vi "Disabled.vi"(11 "Call Context":T1) -> ()   [LabVIEW 2013]
doc: "This VI is called each time a disabled packet is received from the DS. It is often used to prepare for the next robot mode, to calibrate sensors, etc."
uses:
  <vilib>/Rock Robotics/WPI/DriverStation/WPI_DriverStationDerivedRobotMode.ctl
  Robot Global Data.vi
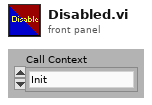
[diagram p1: front panel]
types:
  T1 = typedef "WPI_DriverStationDerivedRobotMode.ctl" = enum16{"Init", "Execute", "Stop"}
  T2 = typedef "Right Drive Joystick.ctl" = cluster{"Buttons":T3, "Axes":cluster{"axis 1 (x)":dbl, "axis 2 (y)":dbl, "axis 3 (throttle)":dbl, "axis 4":dbl, "axis 5":dbl, "axis 6":dbl}}
  T3 = typedef "WPI_JoystickButtonState.ctl" = cluster{"Button 1":bool, "Button 2":bool, "Button 3":bool, "Button 4":bool, "Button 5":bool, "Button 6":bool, "Button 7":bool, "Button 8":bool, "Button 9":bool, "Button 10":bool, "Button 11":bool, "Button 12":bool}
  T4 = typedef "Left Drive Joystick.ctl" = cluster{"Buttons":T3, "Axes":cluster{"axis 1 (x)":dbl, "axis 2 (y)":dbl, "axis 3 (throttle)":dbl, "axis 4":dbl, "axis 5":dbl, "axis 6":dbl}}
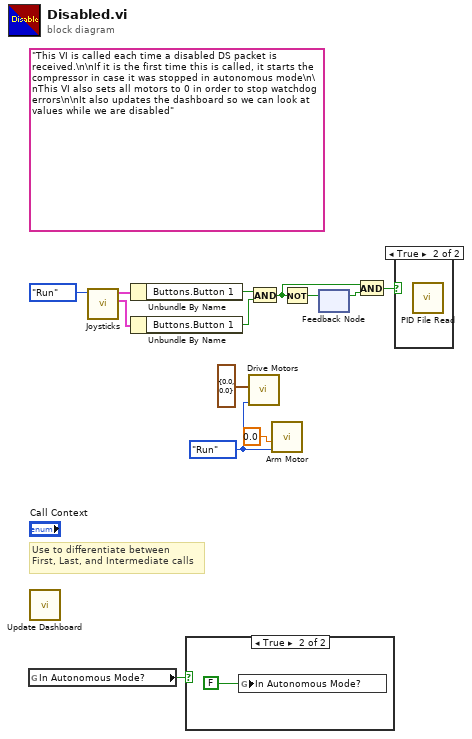
[diagram p0: block diagram]
diagram:
  w10 = enum16{"Init", "Run", "End"}."Run" ("Mode")
  (unwired) "This VI is called each time a disabled DS packet is received.\n\nIf it is the first time this is called, it starts the compressor in case it was stopped in autonomous mode\n\nThis VI also sets all motors to 0 in order to stop watchdog errors\n\nIt also updates the dashboard so we can look at values while we are disabled"
  # "Use to differentiate between\nFirst, Last, and Intermediate calls"
  n1 = global read "Robot Global Data.vi" "In Autonomous Mode?"() -> (w11:bool)
  n2 = call "Update Dashboard.vi"() -> ()  [unwired: 12 out]
  n3 = call "Joysticks.vi"("Mode"=enum16{"Init", "Run", "End"}."Run") -> ("Right Driving Joystick Values"=w7:T2, "Left Driving Joystick Values"=w8:T4)  [unwired: 7 out]
  n4 = Unbundle By Name(w8) -> ("Buttons.Button 1"=w6:bool)
  n5 = Unbundle By Name(w7) -> ("Buttons.Button 1"=w5:bool)
  n6 = case shown="True" w11 {
    frame False {
    }
    frame True {
      n7 = global write "Robot Global Data.vi" "In Autonomous Mode?"(FALSE ("In Autonomous Mode?")) -> ()
    }
  }
  n8 = call "Drive Motors.vi"("Mode"=w10, "Inputs"=cluster{"Left Drive":dbl, "Right Drive":dbl} {"Left Drive"=0.0, "Right Drive"=0.0}) -> ()  [unwired: 1 in, 9 out]
  n9 = And(x=w6, y=w5) -> (x .and. y?=w2:bool)
  n10 = call "Arm Motor.vi"("Mode"=w10, "Arm motor speed"=0.0) -> ()  [unwired: 2 in, 8 out]
  n11 = Not(x=w2) -> (.not. x?=w4:bool)
  n12 = feedback-in #1(w4) -> ()
  n13 = feedback #1() -> (w3:bool)  [unwired: 1 out]
  n14 = And(x=w2, y=w3) -> (x .and. y?=w1:bool)
  n15 = case shown="True" w1 {
    frame False {
    }
    frame True {
      n16 = call "PID File Read.vi"() -> ()  [unwired: 1 out]
    }
  }
